vi "test_ConstructorDefaultValues.vi"() -> (3 "Pass?":bool)   [LabVIEW 2019, in "Tests.SolutionBuilder.lvlib"]
uses:
  Tests.SolutionBuilder.lvlib
  SolutionBuilder/SolutionBuilder.lvclass
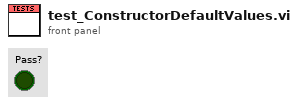
[diagram p1: front panel]
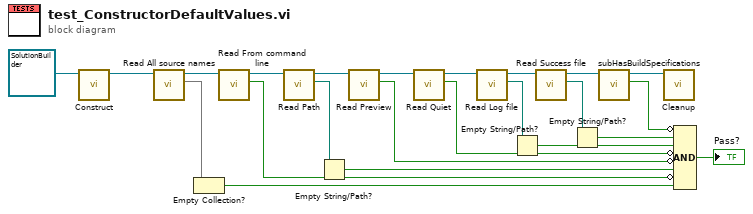
[diagram p0: block diagram]
diagram:
  n1 = call-dynamic "Construct.vi"("SolutionBuilder in"=refnum<class "SolutionBuilder.lvclass"> refnum ("SolutionBuilder.lvlib:SolutionBuilder.lvclass")) -> ("SolutionBuilder out"=w22:refnum<class "SolutionBuilder.lvclass">)  [unwired: 9 in, 1 out]
  n2 = call-dynamic "Read All source names.vi"("SolutionBuilder in"=w22) -> ("All source names"=w17:set{string}, "SolutionBuilder out"=w21:refnum<class "SolutionBuilder.lvclass">)  [unwired: 9 in]
  n3 = Empty Collection?(1:w17) -> (0:w15:bool)
  n4 = call-dynamic "Read From command line.vi"("SolutionBuilder in"=w21) -> ("From command line?"=w14:bool, "SolutionBuilder out"=w20:refnum<class "SolutionBuilder.lvclass">)  [unwired: 9 in]
  n5 = call-dynamic "Read Path.vi"("SolutionBuilder in"=w20) -> ("Path"=w16:path, "SolutionBuilder out"=w19:refnum<class "SolutionBuilder.lvclass">)  [unwired: 9 in]
  n6 = Empty String/Path?(string/path=w16) -> (empty?=w13:bool)
  n7 = call-dynamic "Read Preview.vi"("SolutionBuilder in"=w19) -> ("Preview?"=w12:bool, "SolutionBuilder out"=w18:refnum<class "SolutionBuilder.lvclass">)  [unwired: 9 in]
  n8 = call-dynamic "Read Quiet.vi"("SolutionBuilder in"=w18) -> ("Quiet?"=w11:bool, "SolutionBuilder out"=w7:refnum<class "SolutionBuilder.lvclass">)  [unwired: 9 in]
  n9 = call-dynamic "Read Log file.vi"("SolutionBuilder in"=w7) -> ("Log file"=w2:path, "SolutionBuilder out"=w6:refnum<class "SolutionBuilder.lvclass">)  [unwired: 9 in]
  n10 = Empty String/Path?(string/path=w2) -> (empty?=w3:bool)
  n11 = call-dynamic "Read Success file.vi"("SolutionBuilder in"=w6) -> ("Success file"=w5:path, "SolutionBuilder out"=w1:refnum<class "SolutionBuilder.lvclass">)  [unwired: 9 in]
  n12 = Empty String/Path?(string/path=w5) -> (empty?=w4:bool)
  n13 = call "subHasBuildSpecifications.vi"("SolutionBuilder in"=w1) -> ("Has specs?"=w8:bool, "SolutionBuilder out"=w9:refnum<class "SolutionBuilder.lvclass">)  [unwired: 8 in, 1 out]
  n14 = call-dynamic "Cleanup.vi"("SolutionBuilder in"=w9) -> ()  [unwired: 9 in, 2 out]
  n15 = Compound Arithmetic op=AND(invert w8, w4, w3, invert w11, invert w12, w13, invert w14, w15) -> (→"Pass?":bool)
